vi "Fetch Min Max Waveform.vi"(8 "error in (no error)":errorcluster, 9 "Timeout (10000 ms)":u32=10000, 10 "Source (0: Channel 1)":u16(ring) items=["Channel 1", "Channel 2", "Channel 3", "Channel 4", "Math"], 11 "VISA resource name":refnum<visa-resource-name>) -> (0 "error out":errorcluster, 1 "Min Waveform":waveform(dbl)(graph), 2 "Max Waveform":waveform(dbl)(graph), 3 "VISA resource name out":refnum<visa-resource-name>)   [LabVIEW 2021, in "Agilent 6000 Series.lvlib"]
doc: "Returns the waveform the oscilloscope acquired for the specified channel. The waveform is from an acquisition that you initiate prior to calling this VI.\n\nYou use the Initiate VI to start an acquisition on the channels that you enable with the <B>Configure Channel</B> VI. The oscilloscope acquires waveforms for the enabled channels concurrently. You must call this VI separately for each enabled channel to obtain the waveforms.\n\nYou can call the <B>Read Min Max Waveform</B> VI instead of using low level VIs.\n\n<B>NOTE:</B> \n\n1. This VI should ONLY be used when Acquisition Type is Peak Detect.\n\n2.This VI does not check the instrument status. Typically, you call this VI only in a sequence of calls to other low-level instrument driver VIs. The sequence performs one operation. You use the low-level VIs to optimize one or more aspects of interaction with the instrument."
uses:
  Agilent 6000 Series.lvlib
panel:
  # "NOTE: This VI should ONLY be used when Acquisition Type is Peak Detect"
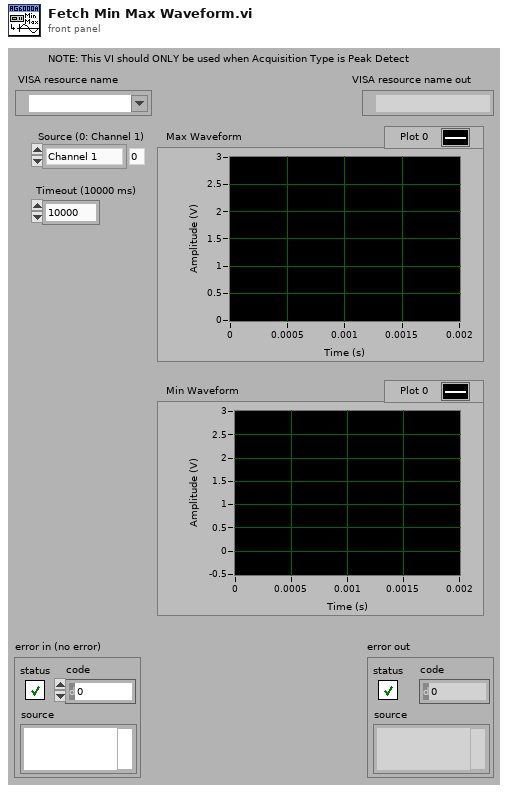
[diagram p1: front panel]
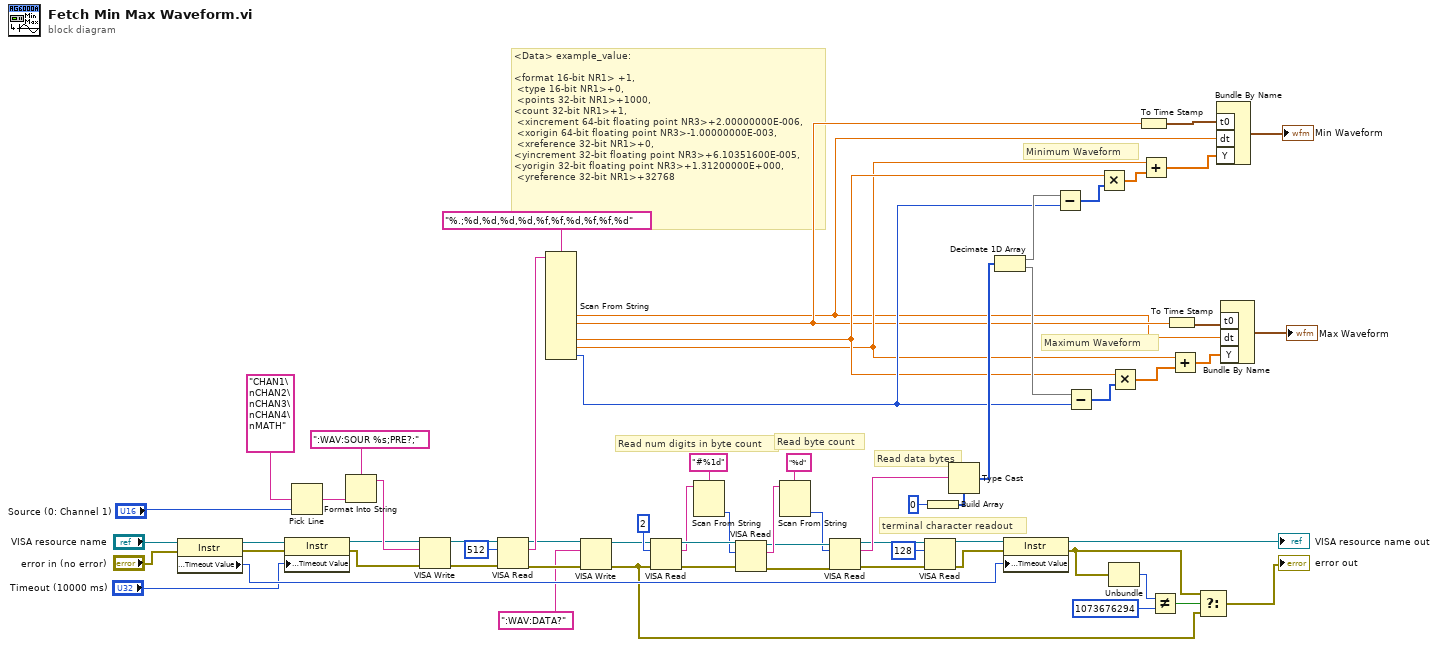
[diagram p0: block diagram]
diagram:
  # "Minimum Waveform"
  # "Maximum Waveform"
  # "<Data> example_value:\n\n<format 16-bit NR1> +1,\n <type 16-bit NR1>+0,\n <points 32-bit NR1>+1000, \n<count 32-bit NR1>+1,\n <xincrement 64-bit floating point NR3>+2.00000000E-006,\n <xorigin 64-bit floating point NR3>-1.00000000E-003,\n <xreference 32-bit NR1>+0, \n<yincrement 32-bit floating point NR3>+6.10351600E-005, \n<yorigin 32-bit floating point NR3>+1.31200000E+000,\n <yreference 32-bit NR1>+32768"
  # "terminal character readout"
  # "Read data bytes"
  # "Read num digits in byte count"
  # "Read byte count"
  n1 = property on="Property Node" class="Instr"(reference="VISA resource name", error in="error in (no error)") -> (reference out=w51:refnum<visa-resource-name>, error out=w50:errorcluster, "General Settings:Timeout Value"=w52:u32)
  n2 = property on="Property Node" class="Instr"(reference=w51, error in=w50, "General Settings:Timeout Value"="Timeout (10000 ms)") -> (reference out=w48:refnum<visa-resource-name>, error out=w47:errorcluster)
  n3 = Pick Line(multi-line string="CHAN1\nCHAN2\nCHAN3\nCHAN4\nMATH", line index="Source (0: Channel 1)") -> (output string=w60:string)  [unwired: 1 in]
  n4 = Format Into String(format string=":WAV:SOUR %s;PRE?;", w60) -> (resulting string=w59:string)  [unwired: 2 in, 1 out]
  n5 = VISA Write(VISA resource name=w48, write buffer=w59, error in (no error)=w47) -> (VISA resource name out=w57:refnum<visa-resource-name>, error out=w58:errorcluster)  [unwired: 1 out]
  n6 = VISA Read(VISA resource name=w57, byte count=u32 512, error in (no error)=w58) -> (VISA resource name out=w46:refnum<visa-resource-name>, read buffer=w55:string, error out=w45:errorcluster)  [unwired: 1 out]
  n7 = Scan From String(format string="%.;%d,%d,%d,%d,%f,%f,%d,%f,%f,%d", input string=w55) -> (output 5=w1:dbl, output 6=w2:dbl, output 8=w5:dbl, output 9=w4:dbl, output 10=w6:i32)  [unwired: 17 in, 3 out]
  n8 = VISA Write(VISA resource name=w46, write buffer=":WAV:DATA?", error in (no error)=w45) -> (VISA resource name out=w37:refnum<visa-resource-name>, error out=w19:errorcluster)  [unwired: 1 out]
  n9 = VISA Read(VISA resource name=w37, byte count=u32 2, error in (no error)=w19) -> (VISA resource name out=w40:refnum<visa-resource-name>, read buffer=w38:string, error out=w41:errorcluster)  [unwired: 1 out]
  n10 = Scan From String(format string="#%1d", input string=w38) -> (output 1=w39:i32)  [unwired: 3 in, 3 out]
  n11 = VISA Read(VISA resource name=w40, byte count=w39, error in (no error)=w41) -> (VISA resource name out=w33:refnum<visa-resource-name>, read buffer=w35:string, error out=w34:errorcluster)  [unwired: 1 out]
  n12 = Scan From String(format string="%d", input string=w35) -> (output 1=w31:i32)  [unwired: 3 in, 3 out]
  n13 = VISA Read(VISA resource name=w33, byte count=w31, error in (no error)=w34) -> (VISA resource name out=w29:refnum<visa-resource-name>, read buffer=w32:string, error out=w30:errorcluster)  [unwired: 1 out]
  n14 = VISA Read(VISA resource name=w29, byte count=u32 128, error in (no error)=w30) -> (VISA resource name out=w28:refnum<visa-resource-name>, error out=w27:errorcluster)  [unwired: 2 out]
  n15 = Build Array(u16 0) -> (w66:u16[])
  n16 = Type Cast(type=w66, x=w32) -> (*(type *) &x=w14:u16[])
  n17 = Decimate 1D Array(w14) -> (w7:u16[], w13:u16[])
  n18 = property on="Property Node" class="Instr"(reference=w28, error in=w27, "General Settings:Timeout Value"=w52) -> (reference out=→"VISA resource name out":refnum<visa-resource-name>, error out=w22:errorcluster)
  n19 = Subtract(x=w7, y=w6) -> (x-y=w9:i32[])
  n20 = Subtract(x=w13, y=w6) -> (x-y=w12:i32[])
  n21 = Multiply(x=w5, y=w9) -> (x*y=w8:dbl[])
  n22 = Unbundle(w22) -> ("code"=w25:i32)  [unwired: 2 out]
  n23 = Multiply(x=w5, y=w12) -> (x*y=w11:dbl[])
  n24 = To Time Stamp(1:w2) -> (0:w16:timestamp)
  n25 = Add(x=w4, y=w8) -> (x+y=w3:dbl[])
  n26 = Not Equal?(x=w25, y=1073676294) -> (x != y?=w23:bool)
  n27 = To Time Stamp(1:w2) -> (0:w18:timestamp)
  n28 = Add(x=w4, y=w11) -> (x+y=w10:dbl[])
  n29 = Select(t=w22, s=w23, f=w19) -> (s? t:f=→"error out":errorcluster)
  n30 = Bundle By Name ("Build Waveform")("t0"=w16, "dt"=w1, "Y"=w3) -> (→"Min Waveform":waveform(dbl))  [unwired: 1 in]
  n31 = Bundle By Name ("Build Waveform")("t0"=w18, "dt"=w1, "Y"=w10) -> (→"Max Waveform":waveform(dbl))  [unwired: 1 in]
